vi "BridgeFun.vi"(11 "Files":T1[](array[typedef])) -> ()   [LabVIEW 2022 SP3]
uses:
  GraphType.ctl
  Curtin1_Label.ctl
panel:
  in  "Task":enum16{"AvR", "AvC"}(ring)
  in  "Bass":string=" B"
  in  "Treble":string=" T"
  out "Sum":cluster{"t0":dbl, "df":dbl, "Y":dbl[]}[](graph)
  in  "zoom":bool
  out "names":string[](array[string])
  in  "Views":T3={"View Type"=0, "Smoothing"=0, "Bands"=0, "Edit"=FALSE, "rescale Y"=FALSE, "rescale X"=FALSE, "X_Low"=0.0, "X_High"=0.0, "dB Range"=40.0, "Excel"=FALSE, "Y Scaling"=FALSE, "X Scaling"=FALSE, "mag/phase 2"=0} {"mag/phase 2" items=["FRF", "rad phase unwrapped", "deg phase unwrapped", "rad phase wrapped", "deg phase wrapped", "White Plots", "MJ Map", "Real and Imaginary"]; "Bands" items=["No Bands", "A Octaves (440-880-1760-3520-7040)", "Curtin Bands (200-780-1740-2930-7000)", "favorites.txt (440)", "JC violin 200-7000 Flat", "JC violin 200-780-1740-2930-7000", "JC violin 200-780-7000", "ObieAlto 200-650-1500-2700-6300 (200-650-1575-2450-6300)"]; "Smoothing" items=["No smoothing"=0, "1/4 semitone"=25, "1/2 semitone"=50, "1 semitone"=100, "2 semitones"=200]; "View Type" items=["As measured"=0, "Normalize"=1, "Cplx Average"=3, "Real Average"=4]}
  out "Difference":cluster{"t0":dbl, "df":dbl, "Y":dbl[]}[](graph)
  # "AvR = RMS average of magnitudes of the complex sum/difference of the position trf files\nAvC = magnitude of the averages of the complex sum/differences of the trf files\n\nI assume that the positions are the same in both cases (001 is the same) and that\nyou have taken the same number of positions"
  # "I assume that the order here is 1,2,3... for B (or T) \nso I subtract the first B from the first T and so on."
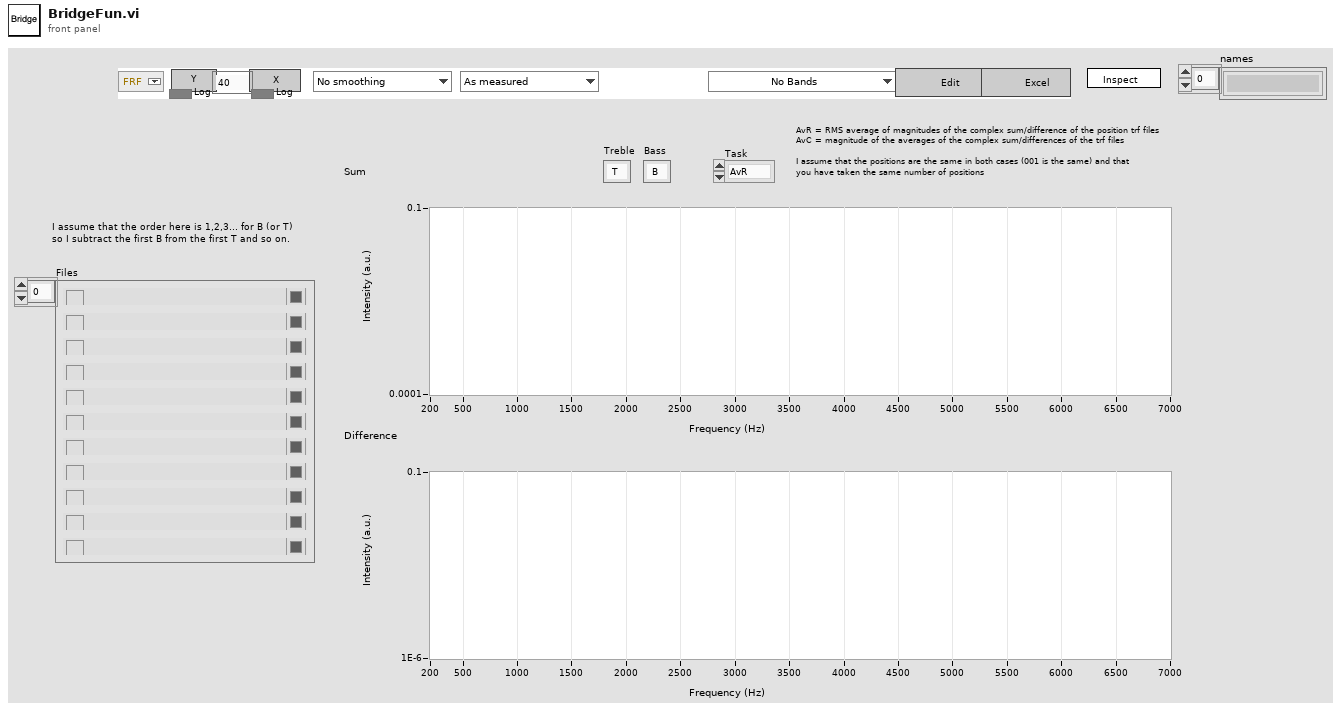
[diagram p1: front panel]
types:
  T1 = typedef "Curtin1_Label.ctl" = cluster{"Show?":bool, "Name":string, "Color":u32, "Path":path, "Show Notes":bool}
  T2 = typedef "GraphType.ctl" = u16
  T3 = cluster{"View Type":u16, "Smoothing":u16, "Bands":u16, "Edit":bool, "rescale Y":bool, "rescale X":bool, "X_Low":dbl, "X_High":dbl, "dB Range":dbl, "Excel":bool, "Y Scaling":bool, "X Scaling":bool, "mag/phase 2":T2}
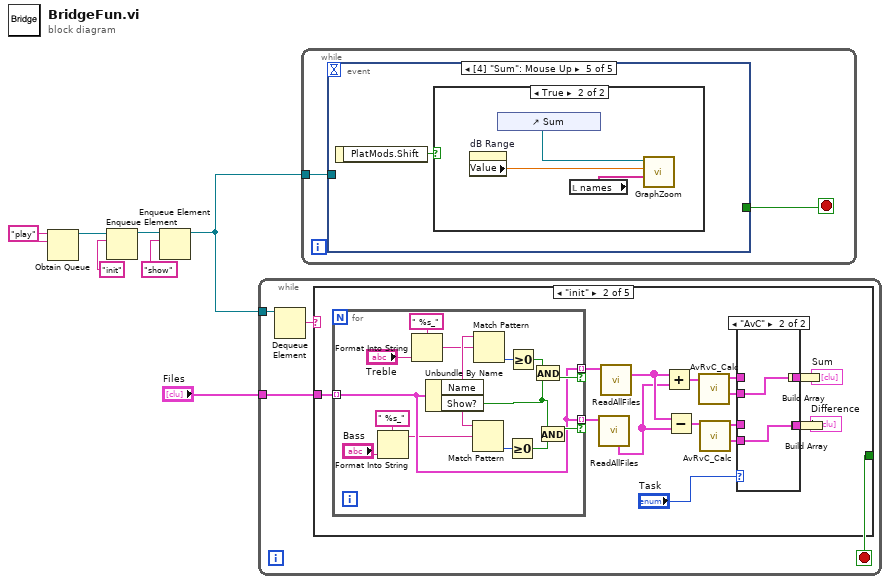
[diagram p0: block diagram]
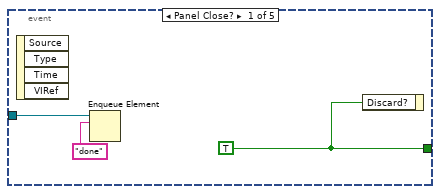
[diagram p2: hidden frame]
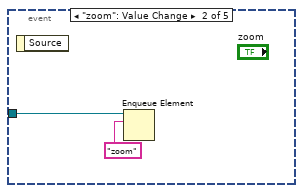
[diagram p3: hidden frame]
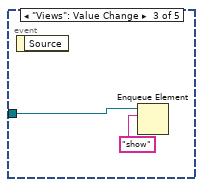
[diagram p4: hidden frame]
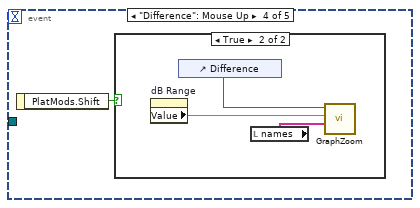
[diagram p5: hidden frame]
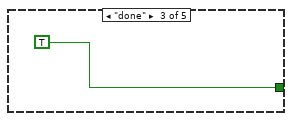
[diagram p10: hidden frame]
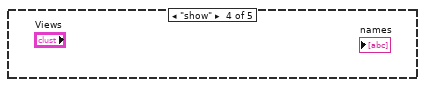
[diagram p11: hidden frame]
diagram:
  w7 = "play" ("name (unnamed)")
  n1 = Obtain Queue(name (unnamed)=w7, element data type=w7) -> (queue out=w2:refnum<queue>)  [unwired: 3 in, 2 out]
  n2 = Enqueue Element(queue=w2, element="init") -> (queue out=w1:refnum<queue>)  [unwired: 2 in, 2 out]
  n3 = Enqueue Element(queue=w1, element="show") -> (queue out=w5:refnum<queue>)  [unwired: 2 in, 2 out]
  n4 = while {
    tunnel: w5 -> [w11]
    tunnel: "Files" -> [w8]
    stop <- w9 stop-if-true
    n5 = Dequeue Element(queue=w11) -> (element=w10:string)  [unwired: 2 in, 3 out]
    n6 = case shown="\"init\"" w10 {
      tunnel: [_ _ TRUE _ _] -> w9
      tunnel: w8 -> [_ w27 _ _ _]
      frame Default {
      }
      frame "init" {
        n7 = for {
          tunnel: w27 -> [w38] mode=indexing
          tunnel: [w38] -> w25 mode=indexing if=w44
          tunnel: [w38] -> w26 mode=indexing if=w39
          n8 = Format Into String(format string=" %s_", "Bass") -> (resulting string=w32:string)  [unwired: 2 in, 1 out]
          n9 = Format Into String(format string=" %s_", "Treble") -> (resulting string=w36:string)  [unwired: 2 in, 1 out]
          n10 = Unbundle By Name(w38) -> ("Name"=w40:string, "Show?"=w41:bool)
          n11 = Match Pattern(string=w40, regular expression=w32) -> (offset past match=w43:i32)  [unwired: 1 in, 3 out]
          n12 = Match Pattern(string=w40, regular expression=w36) -> (offset past match=w46:i32)  [unwired: 1 in, 3 out]
          n13 = Greater Or Equal To 0?(x=w43) -> (x >= 0?=w42:bool)
          n14 = Greater Or Equal To 0?(x=w46) -> (x >= 0?=w45:bool)
          n15 = And(x=w45, y=w41) -> (x .and. y?=w44:bool)
          n16 = And(x=w41, y=w42) -> (x .and. y?=w39:bool)
        }
        n17 = call "ReadAllFiles.vi"("Files"=w26) -> ("data"=w23:cluster{"t0":dbl, "df":dbl, "Y":cdb[]}[])  [unwired: 5 in, 5 out]
        n18 = call "ReadAllFiles.vi"("Files"=w25) -> ("data"=w24:cluster{"t0":dbl, "df":dbl, "Y":cdb[]}[])  [unwired: 5 in, 5 out]
        n19 = Add(x=w24, y=w23) -> (x+y=w21:cluster{"t0":dbl, "df":dbl, "Y":cdb[]}[])
        n20 = Subtract(x=w24, y=w23) -> (x-y=w18:cluster{"t0":dbl, "df":dbl, "Y":cdb[]}[])
        n21 = call "AvRvC_Calc.vi"("data"=w21) -> ("AvC"=w19:cluster{"t0":dbl, "df":dbl, "Y":dbl[]}, "AvR"=w15:cluster{"t0":dbl, "df":dbl, "Y":dbl[]})  [unwired: 9 in]
        n22 = call "AvRvC_Calc.vi"("data"=w18) -> ("AvC"=w16:cluster{"t0":dbl, "df":dbl, "Y":dbl[]}, "AvR"=w14:cluster{"t0":dbl, "df":dbl, "Y":dbl[]})  [unwired: 9 in]
        n23 = case shown="\"AvC\"" "Task" {
          tunnel: [w29 w31] -> w20
          tunnel: w19 -> [_ w31]
          tunnel: [w28 w30] -> w17
          tunnel: w16 -> [_ w30]
          tunnel: w15 -> [w29 _]
          tunnel: w14 -> [w28 _]
          frame "AvR", Default {
          }
          frame "AvC" {
          }
        }
        n24 = Build Array(w20) -> (→"Sum":cluster{"t0":dbl, "df":dbl, "Y":dbl[]}[])
        n25 = Build Array(w17) -> (→"Difference":cluster{"t0":dbl, "df":dbl, "Y":dbl[]}[])
      }
      frame "done" {
      }
      frame "show" {
      }
      frame "zoom" {
      }
    }
  }
  n26 = while {
    tunnel: w5 -> [w48]
    stop <- w49 stop-if-true
    n27 = event shown="[4] \"Sum\": Mouse Up" {
      selector: _ -> [_ _ _ _ _]
      dyn-events: _ -> [_ _ _ _ _]
      timeout: _ -> [_ _ _ _ _]
      tunnel: [w50 _ _ _ _] -> w49
      tunnel: w48 -> [w51 w53 w55 _ _]
      event Panel Close? {
        w50 = TRUE
        n28 = event-data() -> ()  [unwired: 1 in, 4 out]
        n29 = Enqueue Element(queue=w51, element="done") -> ()  [unwired: 2 in, 3 out]
        n30 = event-data("Discard?"=w50) -> ()  [unwired: 1 in, 1 out]
      }
      event "zoom": Value Change {
        n31 = event-data() -> ()  [unwired: 1 in, 1 out]
        n32 = Enqueue Element(queue=w53, element="zoom") -> ()  [unwired: 2 in, 3 out]
      }
      event "Views": Value Change {
        n33 = event-data() -> ()  [unwired: 1 in, 1 out]
        n34 = Enqueue Element(queue=w55, element="show") -> ()  [unwired: 2 in, 3 out]
      }
      event "Difference": Mouse Up {
        n35 = event-data() -> ("PlatMods.Shift"=w57:bool)  [unwired: 1 in]
        n36 = case shown="True" w57 {
          frame False {
          }
          frame True {
            n37 = property on="dB Range" class="DigNum (strict)"() -> ("Value"=w59:dbl)  [unwired: 2 in, 2 out]
            n38 = control-ref of="Difference"() -> (w60:refnum<vi>)
            n39 = local read "names"() -> (w58:string[])
            n40 = call "GraphZoom.vi"("Names"=w58, "dB Range"=w59, "Graph"=w60) -> ()  [unwired: 9 in]
          }
        }
      }
      event "Sum": Mouse Up {
        n41 = event-data() -> ("PlatMods.Shift"=w61:bool)  [unwired: 1 in]
        n42 = case shown="True" w61 {
          frame False {
          }
          frame True {
            n43 = property on="dB Range" class="DigNum (strict)"() -> ("Value"=w63:dbl)  [unwired: 2 in, 2 out]
            n44 = control-ref of="Sum"() -> (w64:refnum<vi>)
            n45 = local read "names"() -> (w62:string[])
            n46 = call "GraphZoom.vi"("Names"=w62, "dB Range"=w63, "Graph"=w64) -> ()  [unwired: 9 in]
          }
        }
      }
    }
  }
